vi "LA_data_decode_Rev02.vi"(10 "Data In":u8[](array[numeric])) -> (1 "Data Packs":dbl, 2 "Data Bytes":dbl, 3 "RG14":u8[](array[numeric]), 5 "All data":u8[](array[numeric]))   [LabVIEW 2012]
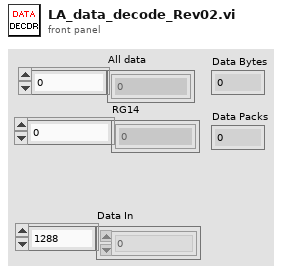
[diagram p1: front panel]
types:
  T1 = cluster{"Boolean array[0]":bool, "Boolean array[1]":bool, "Boolean array[2]":bool, "Boolean array[3]":bool, "Boolean array[4]":bool, "Boolean array[5]":bool, "Boolean array[6]":bool, "Boolean array[7]":bool}
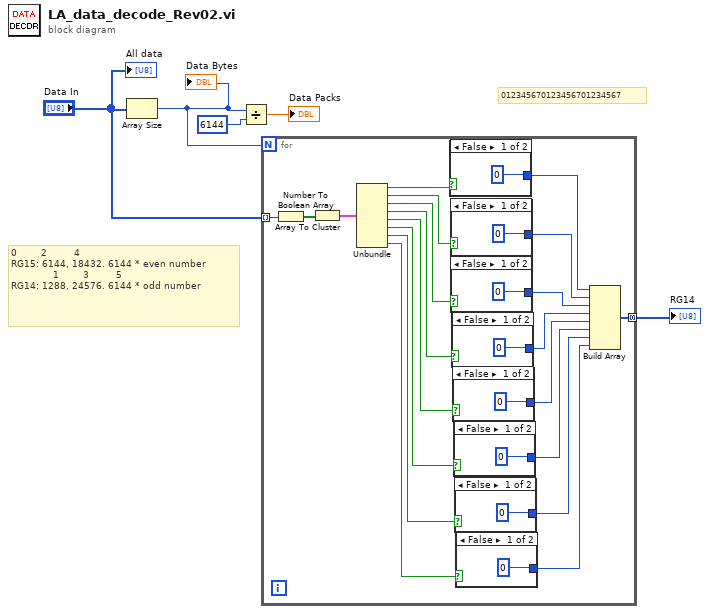
[diagram p0: block diagram]
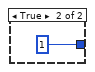
[diagram p2: hidden frame]
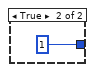
[diagram p3: hidden frame]
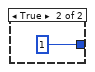
[diagram p4: hidden frame]
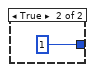
[diagram p5: hidden frame]
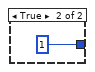
[diagram p6: hidden frame]
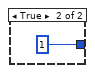
[diagram p7: hidden frame]
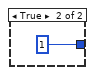
[diagram p8: hidden frame]
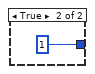
[diagram p9: hidden frame]
diagram:
  # "012345670123456701234567"
  # "0        2         4\nRG15: 6144, 18432. 6144 * even number\n              1        3         5\nRG14: 1288, 24576. 6144 * odd number"
  n1 = Array Size(array="Data In") -> (size(s)=w3:i32)
  "Data Bytes" <- w3
  n2 = Divide(x=w3, y=6144) -> (x/y=→"Data Packs":dbl)
  n3 = for {
    N: w3 -> [_]
    tunnel: "Data In" -> [w25] mode=indexing
    tunnel: [w14] -> w1 mode=concatenating
    n4 = Number To Boolean Array(number=w25) -> (Boolean array=w23:bool[])
    n5 = Array To Cluster(array=w23) -> (cluster=w24:T1)
    n6 = Unbundle(w24) -> ("Boolean array[0]"=w22:bool, "Boolean array[1]"=w21:bool, "Boolean array[2]"=w20:bool, "Boolean array[3]"=w19:bool, "Boolean array[4]"=w18:bool, "Boolean array[5]"=w17:bool, "Boolean array[6]"=w16:bool, "Boolean array[7]"=w15:bool)
    n7 = case shown="False" w22 {
      tunnel: [0 1] -> w13
      frame False {
      }
      frame True {
      }
    }
    n8 = case shown="False" w21 {
      tunnel: [0 1] -> w12
      frame False {
      }
      frame True {
      }
    }
    n9 = case shown="False" w20 {
      tunnel: [0 1] -> w11
      frame False {
      }
      frame True {
      }
    }
    n10 = case shown="False" w19 {
      tunnel: [0 1] -> w10
      frame False {
      }
      frame True {
      }
    }
    n11 = case shown="False" w18 {
      tunnel: [0 1] -> w9
      frame False {
      }
      frame True {
      }
    }
    n12 = case shown="False" w17 {
      tunnel: [0 1] -> w8
      frame False {
      }
      frame True {
      }
    }
    n13 = case shown="False" w16 {
      tunnel: [0 1] -> w7
      frame False {
      }
      frame True {
      }
    }
    n14 = case shown="False" w15 {
      tunnel: [0 1] -> w6
      frame False {
      }
      frame True {
      }
    }
    n15 = Build Array(w13, w12, w11, w10, w9, w8, w7, w6) -> (w14:i32[])
  }
  "RG14" <- w1
  "All data" <- "Data In"
